vi "execution class name.vi"(8 "error in":errorcluster, 11 "TEC configuration in":refnum<class "TEC configuration.lvclass">) -> (0 "error out":errorcluster, 2 "class name":string, 3 "TEC configuration out":refnum<class "TEC configuration.lvclass">)   [LabVIEW 2013, in "TEC configuration.lvclass"]
doc: "Provides an interface for determining the module runtime class associated with this module configuration. This class name can then be used to dynamically load or locate the runtime class for initialization purposes."
uses:
  TEC configuration.lvclass
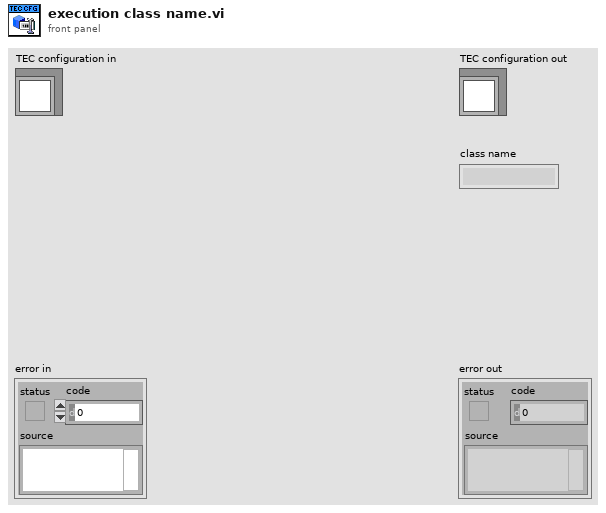
[diagram p1: front panel]
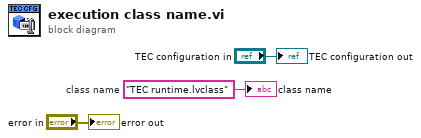
[diagram p0: block diagram]
diagram:
  w1 = "TEC runtime.lvclass"  # class name
  "error out" <- "error in"
  "TEC configuration out" <- "TEC configuration in"
  "class name" <- w1
